vi "YoYoRead.vi"(2 "V/in":dbl=0.098 format="%#_13g", 3 "YoYoDevRef":T1={"DevStatus"={"status"=FALSE, "code"=0, "source"=""}, "Analog Channel"=enum."Invalid"}) -> (0 "YoYo":dbl, 1 "In_Range?":bool)   [LabVIEW 2016, in "ArgosLib.lvlib"]
uses:
  ArgosLib.lvlib
  <vilib>/Rock Robotics/WPI/AnalogChannel/WPI_AnalogChannelDevRef.ctl
  <vilib>/Rock Robotics/SystemInterfaces/AI/FPGA_AIChannel.ctl
panel:
  out "Waveform Chart":cluster{dbl, "Out":dbl}(graph)
  in  "YoYo_Filter_Percent":dbl=0.8
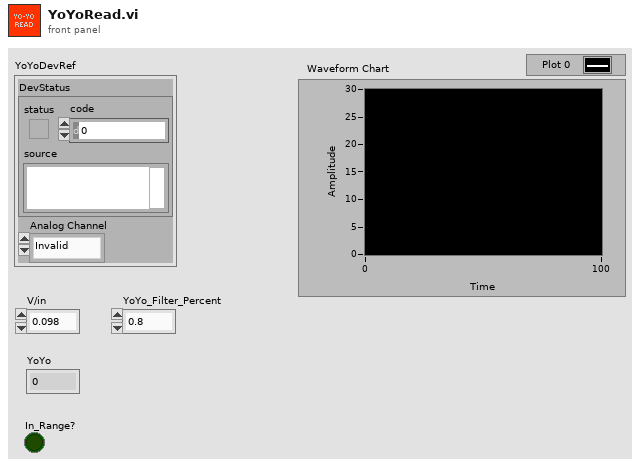
[diagram p1: front panel]
types:
  T1 = typedef "WPI_AnalogChannelDevRef.ctl" = cluster{"DevStatus":errorcluster, "Analog Channel":T2}
  T2 = typedef "FPGA_AIChannel.ctl" = enum8{"AI 0", "AI 1", "AI 2", "AI 3", "AI MXP 0", "AI MXP 1", "AI MXP 2", "AI MXP 3", "Invalid"}
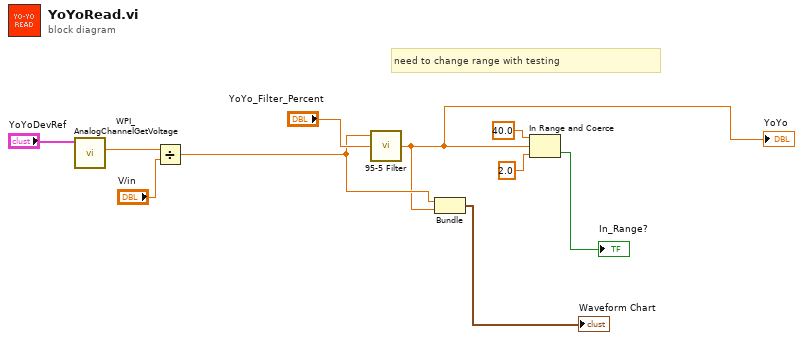
[diagram p0: block diagram]
diagram:
  # "need to change range with testing"
  n1 = call <vilib>:"WPI_AnalogChannelGetVoltage.vi"("AIDeviceRef"="YoYoDevRef") -> ("Voltage"=w9:dbl)  [unwired: 8 in, 2 out]
  n2 = Divide(x=w9, y="V/in") -> (x/y=w3:dbl)
  n3 = call "95-5 Filter.vi"("Percent"="YoYo_Filter_Percent", "In"=w3) -> ("Out"=w2:dbl)  [unwired: 1 in]
  "YoYo" <- w2
  n4 = Bundle(w3, "Out"=w2) -> (→"Waveform Chart":cluster{dbl, "Out":dbl})  [unwired: 1 in]
  n5 = In Range and Coerce(upper limit=40.0, x=w2, lower limit=2.0) -> (In Range?=→"In_Range?":bool)  [unwired: 1 out]
